vi "Creator Queue Alias.vi"(7 "jettl in":refnum<class "jettl.lvclass">, 10 "Queue Mailbox":refnum<data-value>) -> (2 "Creator Queue Alias":string, 5 "jettl out":refnum<class "jettl.lvclass">)   [LabVIEW 2021, in "jettl.lvlib" / "Queue Mailbox.lvlib"]
uses:
  Queue Mailbox.lvlib
  jettl/jettl.lvclass
  Queue Mailbox/Queue Mailbox.lvclass
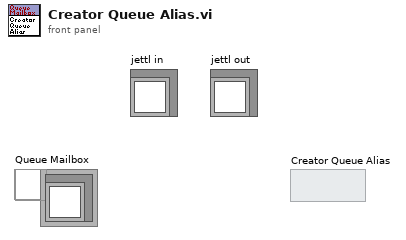
[diagram p1: front panel]
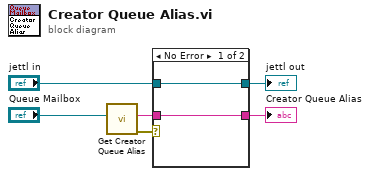
[diagram p0: block diagram]
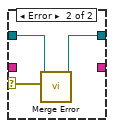
[diagram p2: hidden frame]
diagram:
  n1 = call "Get Creator Queue Alias.vi"("Queue Mailbox"="Queue Mailbox") -> ("error out"=w3:errorcluster, "Creator Queue Alias"=w4:string)  [unwired: 9 in]
  n2 = case shown="No Error" w3 {
    selector: w3 -> [_ w9]
    tunnel: w4 -> [w7 _]
    tunnel: "jettl in" -> [w8 w11]
    tunnel: [w8 w10] -> w5
    tunnel: [w7 _] -> w1
    frame No Error {
    }
    frame Error {
      n3 = call-dynamic "Merge Error.vi"("Error"=w9, "Merge Error in"=w11) -> ("Merge Error out"=w10:refnum<class "jettl.lvclass">)  [unwired: 9 in]
    }
  }
  "jettl out" <- w5
  "Creator Queue Alias" <- w1
